vi "Main.vi"   [LabVIEW 2017]
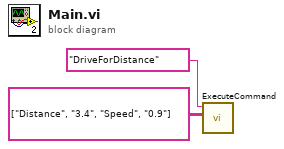
[diagram p0: block diagram]
diagram:
  n1 = call "ExecuteCommand.vi"("Params"=string[][] [["Distance", "3.4"], ["Speed", "0.9"]], "Command"="DriveForDistance") -> ()  [unwired: 10 in]
